vi "AFG3352X.close.vi"(0 "i ref in":refnum<vi>, 3 "ms timeout (10000)":i32=10000, 5 "error in (no error)":errorcluster) -> (14 "i ref out":refnum<vi>, 17 "timed out":bool, 19 "error out":errorcluster)   [LabVIEW 2014, in "AFG3352X.lvlib"]
doc: "Closes the interface to the device."
uses:
  AFG3352X.lvlib
  CSCore/CSApplicationBaseClasses/DeviceBase/DeviceBase.lvlib
  CSinstr.lib/Agilent 3352X Series/Agilent 3352X Series.lvlib
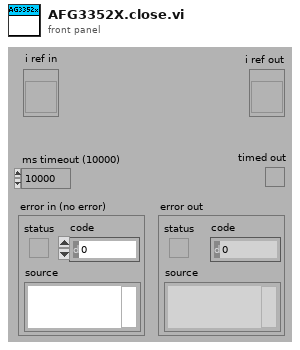
[diagram p1: front panel]
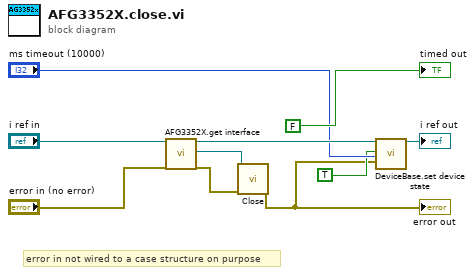
[diagram p0: block diagram]
diagram:
  # "error in not wired to a case structure on purpose"
  n1 = call "AFG3352X.get interface.vi"("i ref in"="i ref in", "error in (no error)"="error in (no error)") -> ("i ref out"=w7:refnum<vi>, "interface"=w2:refnum<visa-resource-name>, "error out"=w3:errorcluster)  [unwired: 15 in]
  n2 = call "Close.vi"("error in (no error)"=w3, "VISA resource name"=w2) -> ("error out"=w1:errorcluster)  [unwired: 9 in]
  "error out" <- w1
  n3 = call "DeviceBase.set device state.vi"("i ref in"=w7, "implicit"=TRUE, "ms timeout (10000)"="ms timeout (10000)", "device error"=w1) -> ("i ref out"=→"i ref out":refnum<vi>)  [unwired: 13 in, 2 out]
  "timed out" <- FALSE
